vi "Init Close.vi"(11 "Test Case In":refnum<class "PCAN Tests.lvclass">) -> (0 "error out":errorcluster, 3 "Test Case Out":refnum<class "PCAN Tests.lvclass">)   [LabVIEW 2025, in "PCAN Tests.lvclass"]
uses:
  PCAN Tests.lvclass
  C:/Program Files/National Instruments/LabVIEW 2025/vi.lib/Astemes/LUnit/Test Case.lvclass
  <vilib>/Astemes/LUnit/Test Case.lvclass/Test Case.ctl
  <vilib>/Astemes/LUnit/Append Pass Result.vi
  <vilib>/Astemes/LUnit/Append Fail Result.vi
  4993e8ee-a06a-463a-9684-69129f64d5ce.vi/9c5d11cd-9439-4240-a1ee-d9baace9c924.vi
  <vilib>/Astemes/LUnit/Run In UI.vi
  <vilib>/Utility/error.llb/Clear Errors.vi
  PCAN Tests.lvclass/PCAN Tests.ctl
  PCAN.lvclass
  <vilib>/Astemes/LUnit/Test Case.lvclass
  C:/Program Files/National Instruments/LabVIEW 2025/vi.lib/Astemes/LUnit/LUnit Runnable.lvclass
  C:/Users/tupp_js/Documents/LabVIEW Data/HAL/source/Devices/PCAN/Tests/PCAN Tests/PCAN Tests.lvclass
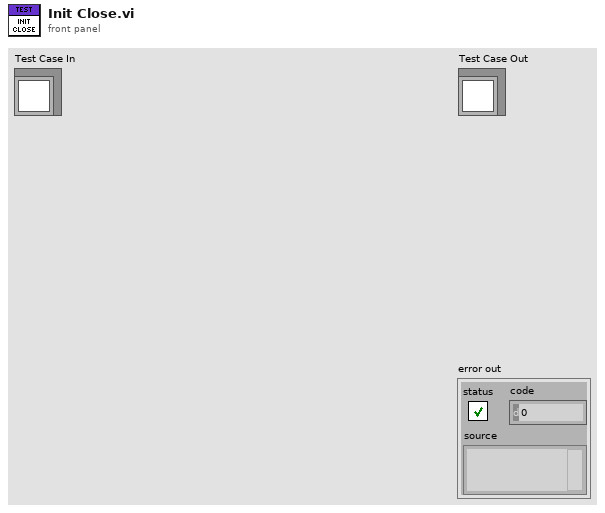
[diagram p1: front panel]
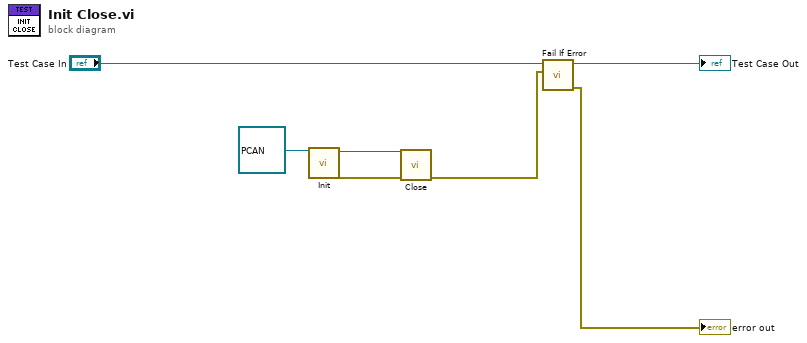
[diagram p0: block diagram]
diagram:
  n1 = call-dynamic "Init.vi"("PCAN in"=refnum<class "PCAN.lvclass"> refnum ("PCAN.lvlib:PCAN.lvclass")) -> ("error out"=w2:errorcluster, "PCAN out"=w3:refnum<class "PCAN.lvclass">)  [unwired: 9 in]
  n2 = call-dynamic "Close.vi"("error in"=w2, "PCAN in"=w3) -> ("error out"=w1:errorcluster)  [unwired: 8 in, 1 out]
  n3 = call <vilib>:"Fail If Error.vi"("Assert error"=w1, "LUnit Test Case In"="Test Case In") -> ("error out"=→"error out":errorcluster, "LUnit Test Case Out"=→"Test Case Out":refnum<class "PCAN Tests.lvclass">)  [unwired: 8 in]
